vi "select rates.vi"(9 "method in":T1={"sampling interval"=0.1, "samples to average"=1, "data interval"=0.0, "stream data"=FALSE, "file path"=refnum, "command"={"command"=enum."Idle", "start time (ms)"=0, "Channel Indices"=[], "Scans per Sample"=1}} {"command"."Scans per Sample" min=1; "data interval" format="%.2f"; "samples to average" min=1 step=1; "sampling interval" format="%.2f"}) -> (3 "method out":T1={"sampling interval"=0.1, "samples to average"=1, "data interval"=0.0, "stream data"=FALSE, "file path"=refnum, "command"={"command"=enum."Idle", "start time (ms)"=0, "Channel Indices"=[], "Scans per Sample"=1}} {"command"."Scans per Sample" min=1; "data interval" format="%.2f"; "samples to average" min=1 step=1; "sampling interval" format="%.2f"}, 6 "sampling rate":dbl format="%.4f", 8 "new samples to average":u32=1 min=1 step=1, 10 "new data interval":sgl format="%.1f", 13 "canceled":bool)   [LabVIEW 2010]
uses:
  DAC apps/support/method.ctl
  DataServer/command cluster.ctl
  DataServer/command.ctl
  DataServer/Server Stats.vi
panel:
  out "Scan rate":dbl=10.0
  out "data rate":sgl format="%.4f"
  in  "rates":T4={"Scans per Sample"=1, "samples to average"=1} {"samples to average" min=1 step=1; "Scans per Sample" min=1}
  in  "cancel":bool
  in  "ok":bool
  # "hz"
  # "hz"
  # "hz"
  # "s"
  # "s"
  # "s"
  # "s"
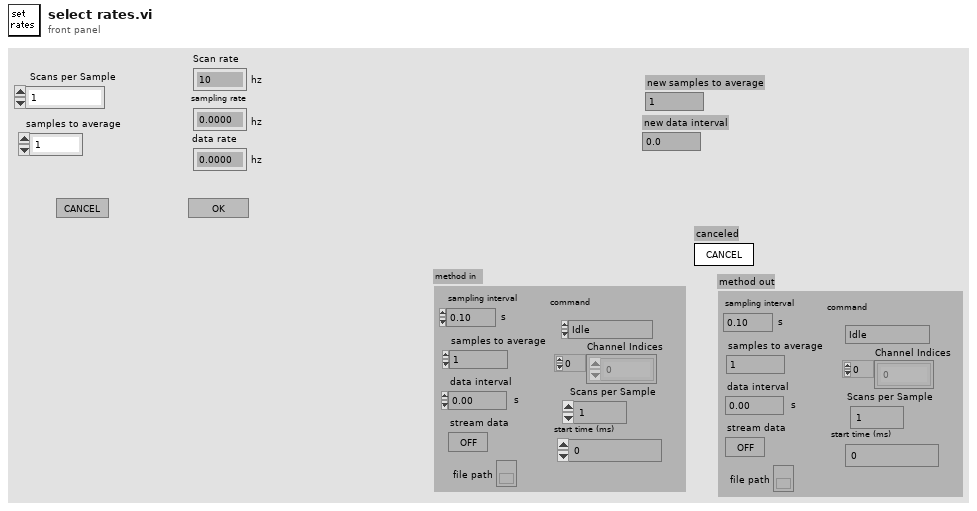
[diagram p1: front panel]
types:
  T1 = typedef "method.ctl" = cluster{"sampling interval":sgl, "samples to average":u32, "data interval":sgl, "stream data":bool, "file path":refnum<file>, "command":T2}
  T2 = typedef "command cluster.ctl" = cluster{"command":T3, "start time (ms)":u32, "Channel Indices":i32[], "Scans per Sample":i32}
  T3 = typedef "command.ctl" = enum16{"Idle", "Send Data", "Send 1 Scan", "Logoff"}
  T4 = cluster{"Scans per Sample":i32, "samples to average":u32}
  T5 = typedef "Server stats.ctl" = cluster{"scan rate":dbl, "# connections":i32, "channel settings":cluster{"Name":string, "upper input limits":sgl, "lower input limits":sgl, "Location":string}[]}
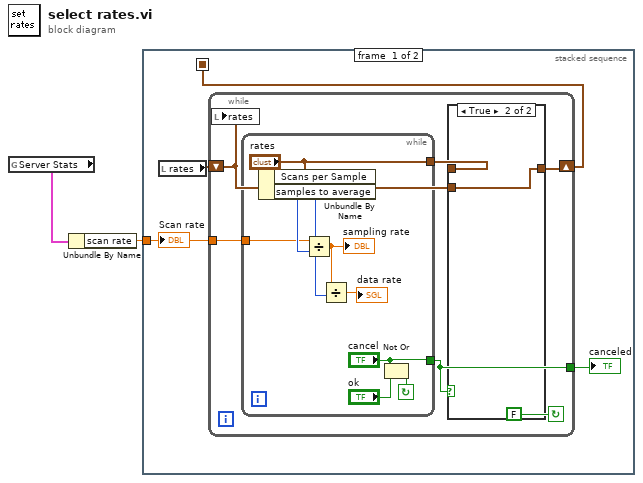
[diagram p0: block diagram]
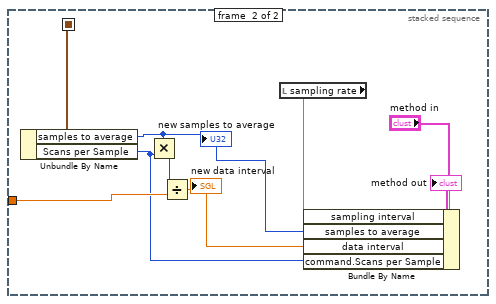
[diagram p3: hidden frame]
diagram:
  n1 = global read "Server Stats.vi" "Server Stats"() -> (w1:T5)
  n2 = Unbundle By Name(w1) -> ("scan rate"=w2:dbl)
  n3 = stacked-sequence {
    seq-local: [w6 _] -> [_ w32]
    tunnel: w2 -> [w3 w27]
    frame #0 {
      n4 = local read "rates"() -> (w4:T4)
      n5 = while {
        tunnel: w3 -> [w8]
        tunnel: [w9] -> w5
        shift-left: w4 -> [w12]
        shift-right: [w11] -> w6
        stop <- FALSE continue-if-true
        n6 = local write "rates"(w12) -> ()
        n7 = while {
          tunnel: w8 -> [w15]
          tunnel: ["cancel"] -> w9
          tunnel: ["rates"] -> w10
          stop <- w20 continue-if-true
          n8 = Unbundle By Name("rates") -> ("Scans per Sample"=w18:i32, "samples to average"=w17:u32)
          n9 = Divide(x=w15, y=w18) -> (x/y=w13:dbl)
          "sampling rate" <- w13
          n10 = Divide(x=w13, y=w17) -> (x/y=→"data rate":dbl)
          n11 = Not Or(1:"ok", 2:"cancel") -> (0:w20:bool)
        }
        n12 = case shown="True" w9 {
          tunnel: [w22 w23] -> w11
          tunnel: w10 -> [w22 _]
          tunnel: w12 -> [_ w23]
          frame False {
          }
          frame True {
          }
        }
      }
      "canceled" <- w5
      "Scan rate" <- w3
    }
    frame #1 {
      n13 = Unbundle By Name(w32) -> ("samples to average"=w26:u32, "Scans per Sample"=w25:i32)
      "new samples to average" <- w26
      n14 = Multiply(x=w26, y=w25) -> (x*y=w24:u32)
      n15 = Divide(x=w24, y=w27) -> (x/y=w31:dbl)
      "new data interval" <- w31
      n16 = local read "sampling rate"() -> (w28:dbl)
      n17 = Bundle By Name(cluster="method in", "sampling interval"=w28, "samples to average"=w26, "data interval"=w31, "command.Scans per Sample"=w25) -> (→"method out":T1)
    }
  }
